vi "Get list of dates.vi"(1 "Year":i32=2021, 2 "Month":i32=4) -> (0 "List":timestamp[](array[timestamp]))   [LabVIEW 2015]
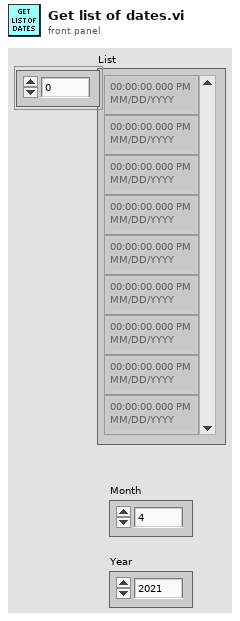
[diagram p1: front panel]
types:
  T1 = typedef "LVDateTimeRec.ctl" = cluster{"fractional second":dbl, "second":i32, "minute":i32, "hour":i32, "day of month":i32, "month":i32, "year":i32, "day of week":i32, "day of year":i32, "DST":i32}
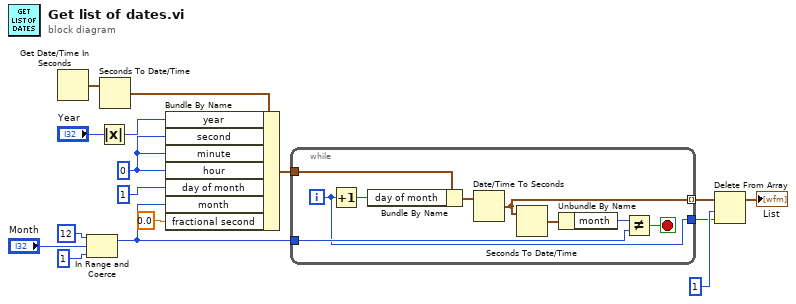
[diagram p0: block diagram]
diagram:
  w14 = 0 ("second")
  n1 = Get Date/Time In Seconds() -> (seconds since 1Jan1904=w16:timestamp)
  n2 = In Range and Coerce(upper limit=12, x="Month", lower limit=1) -> (coerced(x)=w1:i32)  [unwired: 1 out]
  n3 = Absolute Value(x="Year") -> (abs(x)=w5:i32)
  n4 = Seconds To Date/Time(time stamp (now)=w16) -> (date time rec=w15:T1)  [unwired: 1 in]
  n5 = Bundle By Name(cluster=w15, "year"=w5, "second"=w14, "minute"=w14, "hour"=w14, "day of month"=1, "month"=w1, "fractional second"=0.0) -> (w12:T1)
  n6 = while {
    tunnel: w12 -> [w25]
    tunnel: w1 -> [w21]
    tunnel: [w23] -> w11 mode=indexing
    tunnel: [w17] -> w9
    i -> [w17]
    stop <- w19 stop-if-true
    n7 = Increment(x=w17) -> (x+1=w18:i32)
    n8 = Bundle By Name(cluster=w25, "day of month"=w18) -> (w24:T1)
    n9 = Date/Time To Seconds(2:w24) -> (0:w23:timestamp)  [unwired: 1 in]
    n10 = Seconds To Date/Time(time stamp (now)=w23) -> (date time rec=w22:T1)  [unwired: 1 in]
    n11 = Unbundle By Name(w22) -> ("month"=w20:i32)
    n12 = Not Equal?(x=w20, y=w21) -> (x != y?=w19:bool)
  }
  n13 = Delete From Array(array=w11, length=1, index=w9) -> (array with subset deleted=→"List":timestamp[])  [unwired: 1 out]
